vi "Double_ASCII String To Data.vi"(8 "error in (no error)":errorcluster, 9 "Default":dbl, 11 "Value":string) -> (0 "error out":errorcluster, 3 "Data":dbl)   [LabVIEW 2020, in "Current Value Table(Rebuild).lvlib"]
doc: "This VI converts data stored on disk as an ascii string into the correct data type. This VI must perform the opposite operation to the DataToASCIIString function."
uses:
  Current Value Table(Rebuild).lvlib
  Errors/Generate Error.vi
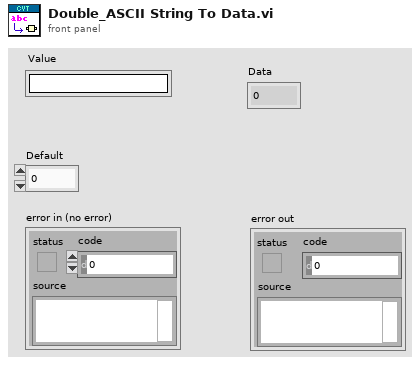
[diagram p1: front panel]
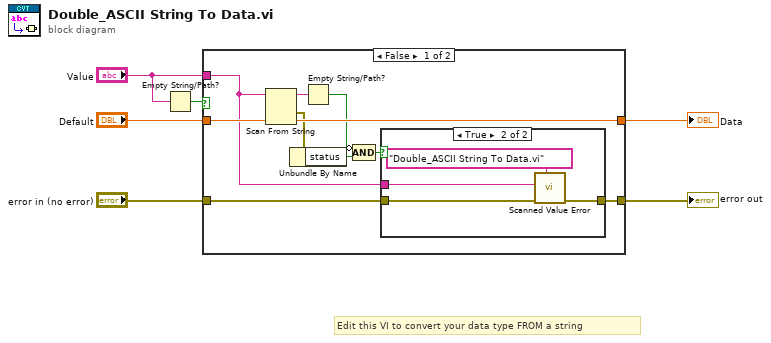
[diagram p0: block diagram]
diagram:
  # "Edit this VI to convert your data type FROM a string"
  n1 = Empty String/Path?(string/path="Value") -> (empty?=w3:bool)
  n2 = case shown="False" w3 {
    tunnel: "Default" -> [w16 w23]
    tunnel: "Value" -> [w8 _]
    tunnel: [w15 w23] -> w1
    tunnel: "error in (no error)" -> [w9 w22]
    tunnel: [w10 w22] -> w5
    frame False {
      n3 = Scan From String(input string=w8, default 1=w16) -> (remaining string=w14:string, error out=w12:errorcluster, output 1=w15:dbl)  [unwired: 3 in, 1 out]
      n4 = Unbundle By Name(w12) -> ("status"=w7:bool)
      n5 = Empty String/Path?(string/path=w14) -> (empty?=w13:bool)
      n6 = Compound Arithmetic op=AND(invert w13, w7) -> (w11:bool)
      n7 = case shown="True" w11 {
        tunnel: [w17 w21] -> w10
        tunnel: w9 -> [w17 w20]
        tunnel: w8 -> [_ w19]
        frame False {
        }
        frame True {
          n8 = call "Scanned Value Error.vi"("caller name"="Double_ASCII String To Data.vi", "error in (no error)"=w20, "Value"=w19) -> ("error out"=w21:errorcluster)  [unwired: 8 in]
        }
      }
    }
    frame True {
    }
  }
  "error out" <- w5
  "Data" <- w1
